vi "solar_read ThisVI.vi"(8 "error in (no error)":errorcluster, 11 "solar in":refnum<class "solar.lvclass">) -> (0 "error out":errorcluster, 2 "VI Refnum":refnum<vi>, 3 "solar out":refnum<class "solar.lvclass">)   [LabVIEW 2018, in "solar.lvclass"]
doc: "This returns this target's VI clone reference."
uses:
  solar.lvclass
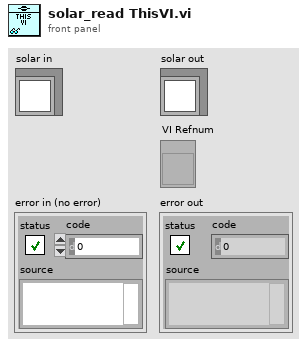
[diagram p1: front panel]
types:
  T1 = typedef "solar_ctl SOLAR Refnum.ctl" = refnum<k1>
  T2 = typedef "solar_ctl SOLAR Global.ctl" = cluster{"Targets":T3[], "AppDir":path, "solar.ini":path, "ConfigsDir":path, "CosmosDir":path, "LogsDir":path, "ExePath":path, "ExeVersion":string, "PartNum":string, "AppSetup":string, "Title":string, "Main.ini":path, "Temp.ini":path, "vSOLAR":string, "Splash.png":string, "SplashWait":i32, "SOLARUE":refnum<user-event>, "VoyagerRefnum":T4, "QTimerRefnum":T5}
  T3 = typedef "solar_ctl Target Global.ctl" = cluster{"Target":string, "Q":refnum<queue>, "UE":refnum<user-event>, "VI":refnum<vi>, "Menu":refnum<k9>, "Data":refnum<data-value>, "Attributes":variant}
  T4 = typedef "solar_voy_ctl Voyager Refnum.ctl" = refnum<k1>
  T5 = typedef "solar_qtimer_ctl Refnum.ctl" = refnum<k1>
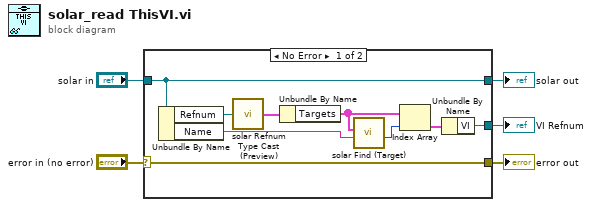
[diagram p0: block diagram]
diagram:
  n1 = case shown="No Error" "error in (no error)" {
    selector: "error in (no error)" -> [w14 w16]
    tunnel: "solar in" -> [w7 w15]
    tunnel: [w14 w16] -> w3
    tunnel: [w7 w15] -> w2
    tunnel: [w6 _] -> w1
    frame No Error {
      n2 = Unbundle By Name(w7) -> ("Refnum"=w10:T1, "Name"=w13:string)
      n3 = call "solar Refnum Type Cast (Preview).vi"("Refnum"=w10) -> ("SOLAR"=w9:T2)  [unwired: 8 in]
      n4 = Unbundle By Name(w9) -> ("Targets"=w11:T3[])
      n5 = call "solar Find (Target).vi"("Target"=w13, "Targets"=w11) -> ("Target Index"=w12:i32)  [unwired: 8 in, 1 out]
      n6 = Index Array(array=w11, index=w12) -> (element=w8:T3)
      n7 = Unbundle By Name(w8) -> ("VI"=w6:refnum<vi>)
    }
    frame Error {
    }
  }
  "error out" <- w3
  "solar out" <- w2
  "VI Refnum" <- w1
